vi "NPL_Simulated Temperature Control with Logging and Stop.vi"(11 "Log File Path":path) -> ()   [LabVIEW 2010]
uses:
  SupportVIs.llb/TS_RT-Open/Create/Replace File.vi
panel:
  in  "TCP port":u16=12344
  in  "error in (no error)":errorcluster
  out "error out":errorcluster
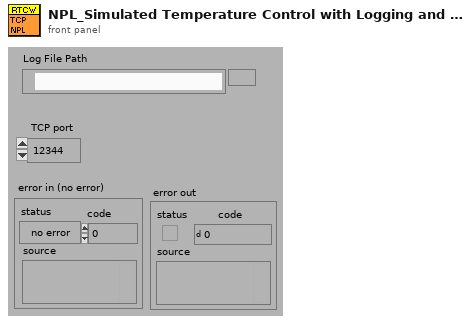
[diagram p1: front panel]
types:
  T1 = enum16{"open", "open or create", "create or replace", "create", "open (read only)"}
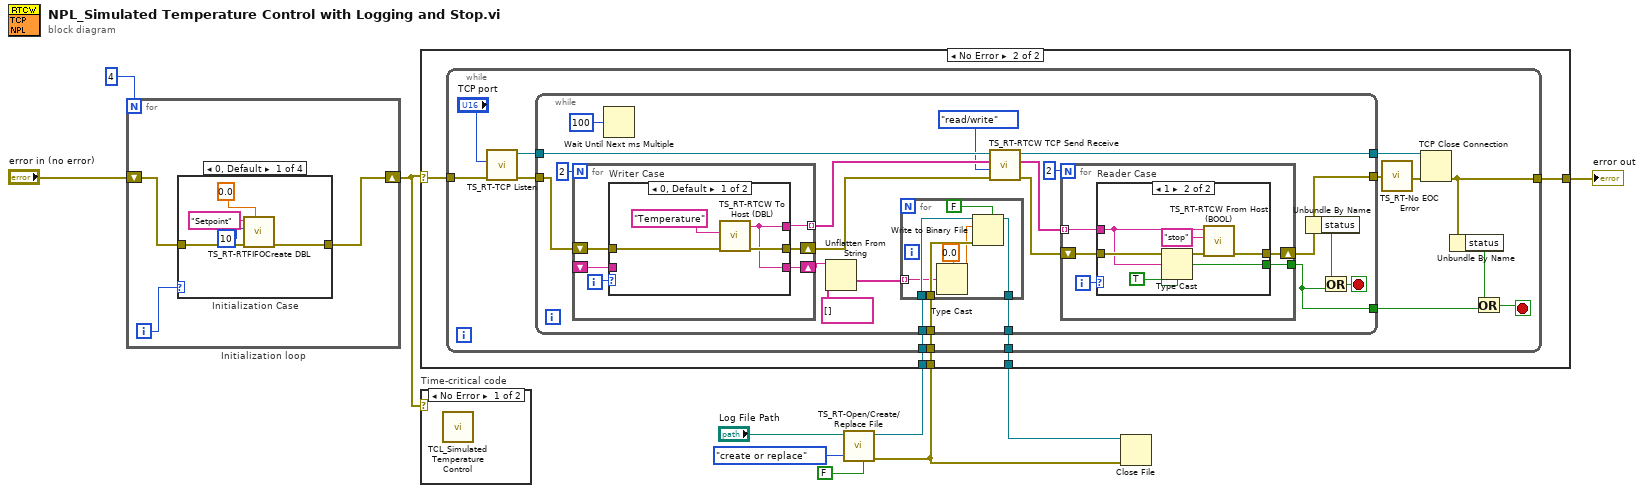
[diagram p0: block diagram]
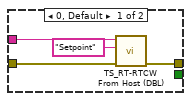
[diagram p4: hidden frame]
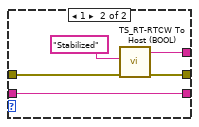
[diagram p5: hidden frame]
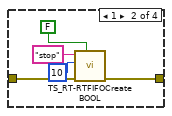
[diagram p6: hidden frame]
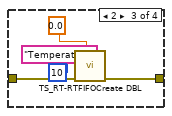
[diagram p7: hidden frame]
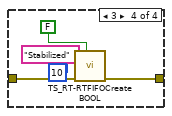
[diagram p8: hidden frame]
diagram:
  n1 = for "Initialization loop" {
    N: 4 -> [_]
    shift-right: [w11] -> w8
    shift-left: "error in (no error)" -> [w12]
    i -> [w13]
    n2 = case "Initialization Case" shown="0, Default" w13 {
      tunnel: w12 -> [w18 w23 w28 w33]
      tunnel: [w17 w22 w27 w32] -> w11
      frame 0, Default {
        n3 = call "TS_RT-RTFIFOCreate DBL.vi"("type"=0.0, "error in (no error)"=w18, "size (10)"=u32 10, "name (unnamed)"="Setpoint") -> ("error out"=w17:errorcluster)  [unwired: 1 in, 6 out]
      }
      frame 1 {
        n4 = call "TS_RT-RTFIFOCreate BOOL.vi"("type"=FALSE, "error in (no error)"=w23, "size (10)"=u32 10, "name (unnamed)"="stop") -> ("error out"=w22:errorcluster)  [unwired: 1 in, 6 out]
      }
      frame 2 {
        n5 = call "TS_RT-RTFIFOCreate DBL.vi"("type"=0.0, "error in (no error)"=w28, "size (10)"=u32 10, "name (unnamed)"="Temperature") -> ("error out"=w27:errorcluster)  [unwired: 1 in, 6 out]
      }
      frame 3 {
        n6 = call "TS_RT-RTFIFOCreate BOOL.vi"("type"=FALSE, "error in (no error)"=w33, "size (10)"=u32 10, "name (unnamed)"="Stabilized") -> ("error out"=w32:errorcluster)  [unwired: 1 in, 6 out]
      }
    }
  }
  n7 = case "Time-critical code" shown="No Error" w8 {
    frame No Error {
      n8 = call "TCL_Simulated Temperature Control.vi"() -> ()  [unwired: 1 out]
    }
    frame Error {
    }
  }
  n9 = call "TS_RT-Open/Create/Replace File.vi"("advisory dialog? (display:T)"=FALSE, "function (open:0)"=T1."create or replace", "file path"="Log File Path") -> ("error out"=w4:errorcluster, "refnum"=w5:refnum<file>)  [unwired: 4 in, 3 out]
  n10 = case shown="No Error" w8 {
    selector: w8 -> [w35 w39]
    tunnel: [w35 w40] -> w10
    tunnel: w5 -> [w34 w38]
    tunnel: w4 -> [_ w37]
    tunnel: [w34 w36] -> w3
    frame Error {
    }
    frame No Error {
      n11 = while "While Loop1" {
        tunnel: [w41] -> w40
        tunnel: w39 -> [w50]
        tunnel: w38 -> [w47]
        tunnel: w37 -> [w46]
        tunnel: [w45] -> w36
        stop <- w43 stop-if-true
        n12 = call "TS_RT-TCP Listen.vi"("error in (no error)"=w50, "port"="TCP port") -> ("error out"=w49:errorcluster, "connection ID"=w52:refnum<k5>)  [unwired: 1 in, 7 out]
        n13 = while "While Loop2" {
          tunnel: w52 -> [w75]
          tunnel: [w74] -> w53
          tunnel: w49 -> [w71]
          tunnel: [w58] -> w48
          tunnel: w47 -> [w62]
          tunnel: w46 -> [w61]
          tunnel: [w60] -> w45
          tunnel: [w55] -> w44
          stop <- w56 stop-if-true
          n14 = for {
            N: 2 -> [_]
            tunnel: [w103] -> w72 mode=indexing
            shift-right: [w100] -> w70
            shift-left: w71 -> [w101]
            shift-right: [w99] -> w64
            shift-left: _ -> [w98]
            i -> [w102]
            n15 = case "Writer Case" shown="0, Default" w102 {
              tunnel: [w104 w110] -> w103
              tunnel: [w106 w111] -> w100
              tunnel: w101 -> [w107 w112]
              tunnel: [w104 w108] -> w99
              tunnel: w98 -> [_ w108]
              frame 0, Default {
                n16 = call "TS_RT-RTCW To Host (DBL).vi"("error in (no error)"=w107, "name (unnamed)"="Temperature") -> ("error out"=w106:errorcluster, "Data"=w104:string)  [unwired: 8 out]
              }
              frame 1 {
                n17 = call "TS_RT-RTCW To Host (BOOL).vi"("error in (no error)"=w112, "name (unnamed)"="Stabilized") -> ("error out"=w111:errorcluster, "Data"=w110:string)  [unwired: 8 out]
              }
            }
          }
          n18 = Wait Until Next ms Multiple(millisecond multiple=u32 100) -> ()  [unwired: 1 out]
          n19 = Unflatten From String(type=string[] [] ("Data Out"), binary string=w64) -> (value=w59:string[])  [unwired: 1 in, 4 out]
          n20 = for {
            tunnel: w62 -> [w82]
            tunnel: [w81] -> w60
            tunnel: w61 -> [w80]
            tunnel: w59 -> [w79] mode=indexing
            n21 = Type Cast(type=0.0, x=w79) -> (*(type *) &x=w77:dbl)
            n22 = Write to Binary File(file (use dialog)=w82, data=w77, error in=w80, 5:FALSE ("prepend array or string size? (T)")) -> (refnum out=w81:refnum<file>)  [unwired: 4 out]
          }
          n23 = call "TS_RT-RTCW TCP Send Receive.vi"("error in (no error)"=w70, "access (read/write)"=enum16{"read/write", "read only", "write only"}."read/write", "Data In"=w72, "connection ID"=w75) -> ("error out"=w69:errorcluster, "Data Out"=w73:string[], "connection ID Out"=w74:refnum<k5>)  [unwired: 1 out]
          n24 = for {
            N: 2 -> [_]
            tunnel: w73 -> [w86] mode=indexing
            shift-right: [w85] -> w58
            shift-left: w69 -> [w84]
            tunnel: [w83] -> w55
            i -> [w87]
            n25 = case "Reader Case" shown="1" w87 {
              tunnel: w84 -> [w90 w96]
              tunnel: [w91 w97] -> w85
              tunnel: w86 -> [w89 w93]
              tunnel: [_ w92] -> w83
              frame 0, Default {
                n26 = call "TS_RT-RTCW From Host (DBL).vi"("error in"=w90, "name (unnamed)"="Setpoint", "Data In"=w89) -> ("error out"=w91:errorcluster)  [unwired: 8 out]
              }
              frame 1 {
                n27 = Type Cast(type=TRUE, x=w93) -> (*(type *) &x=w92:bool)
                n28 = call "TS_RT-RTCW From Host (BOOL).vi"("error in"=w96, "name (unnamed)"="stop", "Data In"=w93) -> ("error out"=w97:errorcluster)  [unwired: 8 out]
              }
            }
          }
          n29 = Unbundle By Name(w58) -> ("status"=w57:bool)
          n30 = Or(x=w57, y=w55) -> (x .or. y?=w56:bool)
        }
        n31 = call "TS_RT-No EOC Error.vi"("error in (no error)"=w48) -> ("error out"=w54:errorcluster)  [unwired: 4 out]
        n32 = TCP Close Connection(connection ID=w53, error in (no error)=w54) -> (error out=w41:errorcluster)  [unwired: 2 out]
        n33 = Unbundle By Name(w41) -> ("status"=w42:bool)
        n34 = Or(x=w42, y=w44) -> (x .or. y?=w43:bool)
      }
    }
  }
  "error out" <- w10
  n35 = Close File(refnum=w3, error in=w4) -> ()  [unwired: 2 out]
